vi "12kW_SubVI.vi"() -> ()   [LabVIEW 2020]
panel:
  out "Step 7\nIndicator":bool
  out "Step 4\nIndicator":bool
  out "Step 10\nIndicator":bool
  out "Step 9\nIndicator":bool
  out "Step 8\nIndicator":bool
  out "Step 6\nIndicator":bool
  out "Step 5\nIndicator":bool
  out "Step 3\nIndicator":bool
  out "Step 2\nIndicator":bool
  out "Step 1\nIndicator":bool
  in  "Stop":bool
  out "Voltage (V)":dbl
  in  "Power Supply":bool
  out "B":bool
  out "Y":bool
  out "R":bool
  out "No. of Resistors Used":i32
  in  "Step Type":enum32{"Variable Steps", "Equal Steps"}(tab)
  in  "Step 1\n250W":bool
  in  "Step 2\n250W":bool
  in  "Step 3\n500W":bool
  in  "Step 4\n1000W":bool
  in  "Step 5\n1000W":bool
  in  "Step 6\n1000W":bool
  in  "Step 7\n2000W":bool
  in  "Step 8\n2000W":bool
  in  "Step 9\n2000W":bool
  in  "Step 10\n2000W":bool
  in  "No. of Equal Steps":T1(tab)
  in  "Step 2\n6000W":bool
  in  "Step 1\n6000W":bool
  in  "Step 3\n4000W":bool
  in  "Step 2\n4000W":bool
  in  "Step 1\n4000W":bool
  in  "Step 4\n3000W":bool
  in  "Step 3\n3000W":bool
  in  "Step 2\n3000W":bool
  in  "Step 1\n3000W":bool
  in  "Step 6\n2000W":bool
  in  "Step 5\n2000W":bool
  in  "Step 4\n2000W":bool
  in  "Step 3\n2000W":bool
  in  "Step 2\n2000W":bool
  in  "Step 1\n2000W":bool
  in  "Master Switch":bool
  out "Load (kW)":dbl
  out "Current (A)":dbl format="%.4f"
  # "Three Phase Variable Resistive Load Bank with 12kW Maximum Capacity and 10 Step Control"
  # "690 ohm\n0.35 A"
  # "All resistors are connected in 3 phase star formation"
  # "690 ohm\n0.35 A"
  # "344 ohm\n0.70 A"
  # "3 Phase Voltage Indicator"
  # "172 ohm\n1.39 A"
  # "172 ohm\n1.39 A"
  # "172 ohm\n1.39 A"
  # "86 ohm\n2.78 A"
  # "86 ohm\n2.78 A"
  # "86 ohm\n2.78 A"
  # "Each Resistor Looks Like This"
  # "86 ohm\n2.78 A"
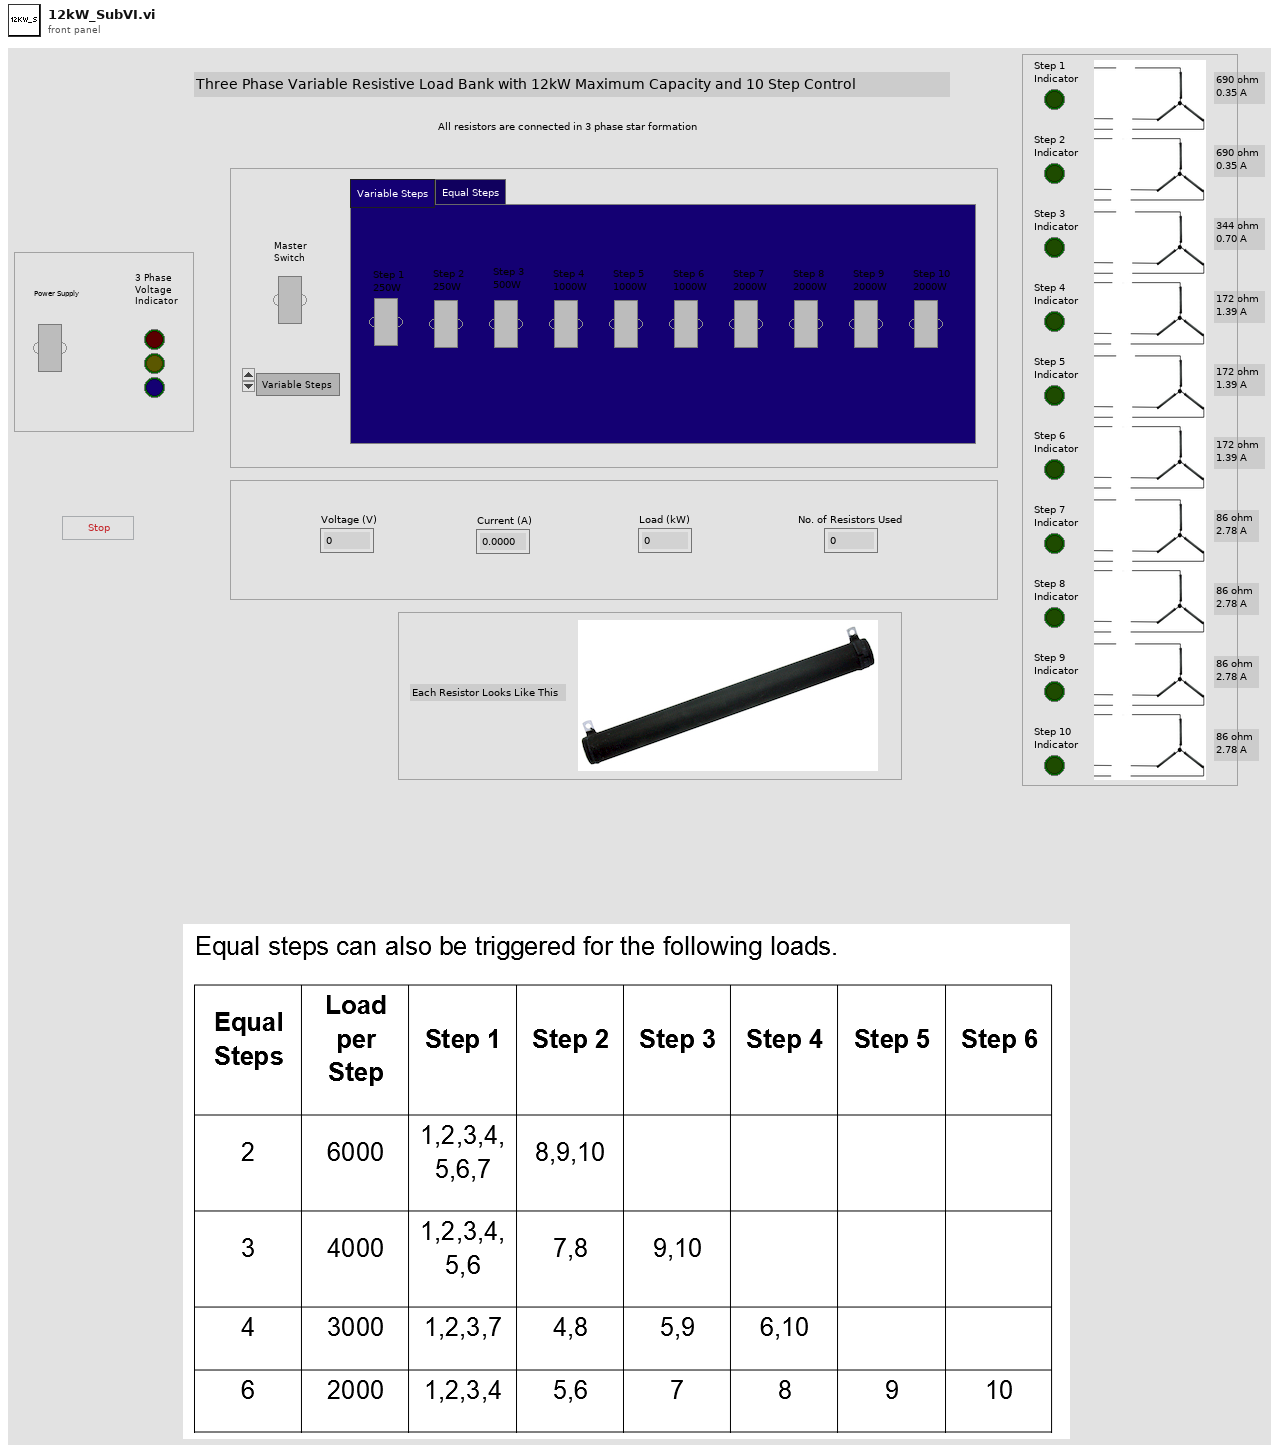
[diagram p1: front panel]
types:
  T1 = enum32{"2 Steps", "3 Steps", "4 Steps", "6 Steps"}
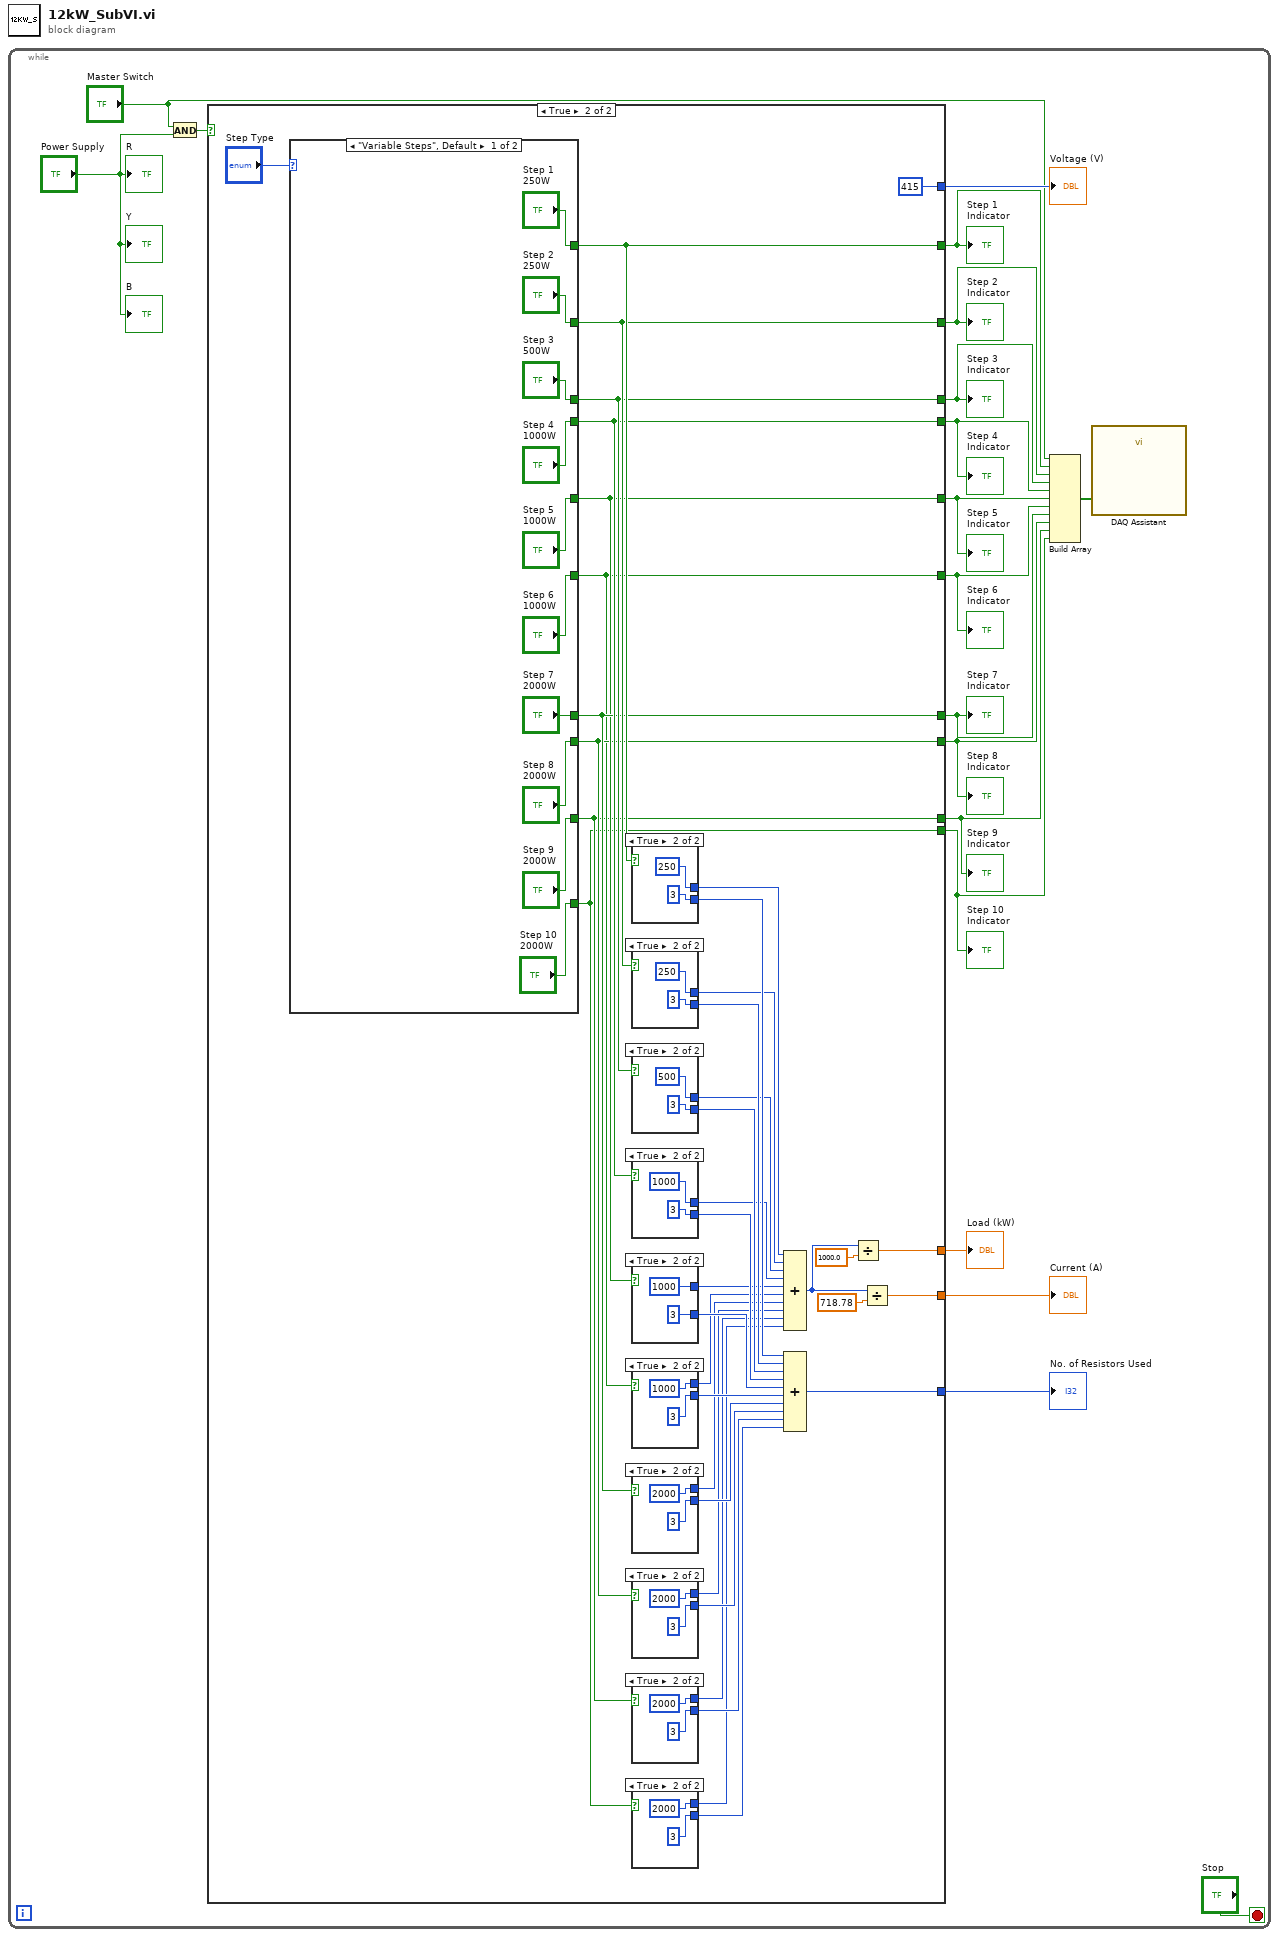
[diagram p0: block diagram]
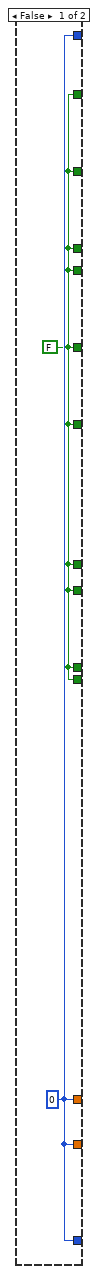
[diagram p2: hidden frame]
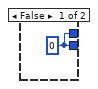
[diagram p3: hidden frame]
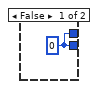
[diagram p4: hidden frame]
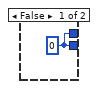
[diagram p5: hidden frame]
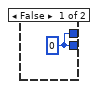
[diagram p6: hidden frame]
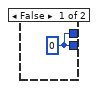
[diagram p7: hidden frame]
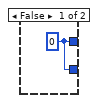
[diagram p8: hidden frame]
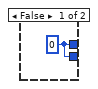
[diagram p9: hidden frame]
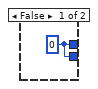
[diagram p10: hidden frame]
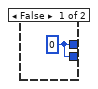
[diagram p11: hidden frame]
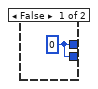
[diagram p12: hidden frame]
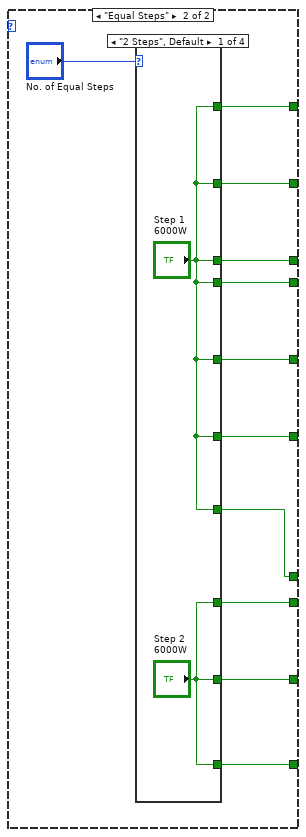
[diagram p13: hidden frame]
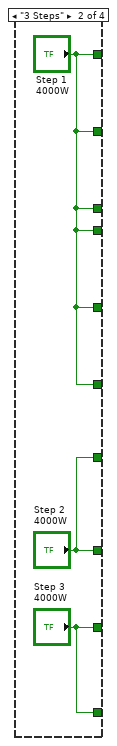
[diagram p14: hidden frame]
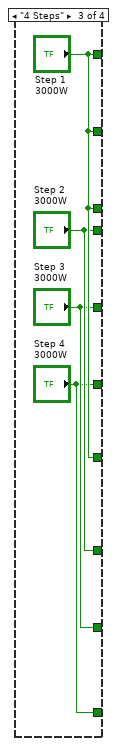
[diagram p15: hidden frame]
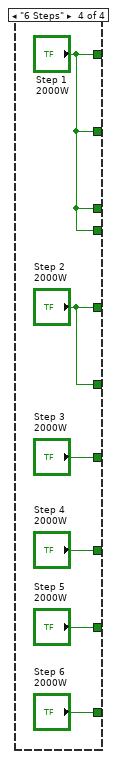
[diagram p16: hidden frame]
diagram:
  n1 = while {
    stop <- "Stop" stop-if-true
    n2 = And(x="Master Switch", y="Power Supply") -> (x .and. y?=w15:bool)
    n3 = case shown="True" w15 {
      tunnel: [w21 w36] -> w18
      tunnel: [w21 w32] -> w17
      tunnel: [w21 w33] -> w19
      tunnel: [w21 415] -> w16
      tunnel: [w20 w31] -> w3
      tunnel: [w20 w30] -> w4
      tunnel: [w20 w29] -> w5
      tunnel: [w20 w28] -> w6
      tunnel: [w20 w27] -> w7
      tunnel: [w20 w26] -> w1
      tunnel: [w20 w25] -> w8
      tunnel: [w20 w24] -> w2
      tunnel: [w20 w23] -> w9
      tunnel: [w20 w22] -> w10
      frame False {
        w20 = FALSE
        w21 = 0
      }
      frame True {
        n4 = case shown="\"Variable Steps\", Default" "Step Type" {
          tunnel: ["Step 10\n2000W" w100] -> w22
          tunnel: ["Step 9\n2000W" w101] -> w23
          tunnel: ["Step 8\n2000W" w102] -> w25
          tunnel: ["Step 7\n2000W" w103] -> w27
          tunnel: ["Step 6\n1000W" w104] -> w24
          tunnel: ["Step 5\n1000W" w105] -> w26
          tunnel: ["Step 4\n1000W" w106] -> w28
          tunnel: ["Step 3\n500W" w107] -> w29
          tunnel: ["Step 2\n250W" w108] -> w30
          tunnel: ["Step 1\n250W" w109] -> w31
          frame "Variable Steps", Default {
          }
          frame "Equal Steps" {
            n5 = case shown="\"2 Steps\", Default" "No. of Equal Steps" {
              tunnel: ["Step 1\n6000W" "Step 1\n4000W" "Step 1\n3000W" "Step 1\n2000W"] -> w109
              tunnel: ["Step 1\n6000W" "Step 1\n4000W" "Step 1\n3000W" "Step 1\n2000W"] -> w108
              tunnel: ["Step 1\n6000W" "Step 1\n4000W" "Step 1\n3000W" "Step 1\n2000W"] -> w107
              tunnel: ["Step 1\n6000W" "Step 1\n4000W" "Step 2\n3000W" "Step 1\n2000W"] -> w106
              tunnel: ["Step 1\n6000W" "Step 1\n4000W" "Step 3\n3000W" "Step 2\n2000W"] -> w105
              tunnel: ["Step 1\n6000W" "Step 1\n4000W" "Step 4\n3000W" "Step 2\n2000W"] -> w104
              tunnel: ["Step 1\n6000W" "Step 2\n4000W" "Step 1\n3000W" "Step 3\n2000W"] -> w103
              tunnel: ["Step 2\n6000W" "Step 2\n4000W" "Step 2\n3000W" "Step 4\n2000W"] -> w102
              tunnel: ["Step 2\n6000W" "Step 3\n4000W" "Step 3\n3000W" "Step 5\n2000W"] -> w101
              tunnel: ["Step 2\n6000W" "Step 3\n4000W" "Step 4\n3000W" "Step 6\n2000W"] -> w100
              frame "2 Steps", Default {
              }
              frame "3 Steps" {
              }
              frame "4 Steps" {
              }
              frame "6 Steps" {
              }
            }
          }
        }
        n6 = case shown="True" w31 {
          tunnel: [w87 250] -> w37
          tunnel: [w87 3] -> w47
          frame False {
            w87 = 0
          }
          frame True {
          }
        }
        n7 = case shown="True" w30 {
          tunnel: [w84 250] -> w38
          tunnel: [w84 3] -> w48
          frame False {
            w84 = 0
          }
          frame True {
          }
        }
        n8 = case shown="True" w29 {
          tunnel: [w81 500] -> w39
          tunnel: [w81 3] -> w49
          frame False {
            w81 = 0
          }
          frame True {
          }
        }
        n9 = case shown="True" w28 {
          tunnel: [w78 1000] -> w40
          tunnel: [w78 3] -> w50
          frame False {
            w78 = 0
          }
          frame True {
          }
        }
        n10 = case shown="True" w26 {
          tunnel: [w75 1000] -> w41
          tunnel: [w75 3] -> w51
          frame False {
            w75 = 0
          }
          frame True {
          }
        }
        n11 = case shown="True" w24 {
          tunnel: [w72 1000] -> w42
          tunnel: [w72 3] -> w52
          frame False {
            w72 = 0
          }
          frame True {
          }
        }
        n12 = case shown="True" w27 {
          tunnel: [w69 2000] -> w43
          tunnel: [w69 3] -> w53
          frame False {
            w69 = 0
          }
          frame True {
          }
        }
        n13 = case shown="True" w25 {
          tunnel: [w66 2000] -> w44
          tunnel: [w66 3] -> w54
          frame False {
            w66 = 0
          }
          frame True {
          }
        }
        n14 = case shown="True" w23 {
          tunnel: [w63 2000] -> w45
          tunnel: [w63 3] -> w55
          frame False {
            w63 = 0
          }
          frame True {
          }
        }
        n15 = case shown="True" w22 {
          tunnel: [w60 2000] -> w46
          tunnel: [w60 3] -> w56
          frame False {
            w60 = 0
          }
          frame True {
          }
        }
        n16 = Compound Arithmetic op=ADD(w37, w38, w39, w40, w41, w42, w43, w44, w45, w46) -> (w35:i32)
        n17 = Compound Arithmetic op=ADD(w47, w48, w49, w50, w51, w52, w53, w54, w55, w56) -> (w36:i32)
        n18 = Divide(x=w35, y=1000.0) -> (x/y=w33:dbl)
        n19 = Divide(x=w35, y=718.78) -> (x/y=w32:dbl)
      }
    }
    "Load (kW)" <- w19
    "Current (A)" <- w17
    "No. of Resistors Used" <- w18
    "Voltage (V)" <- w16
    "Step 1\nIndicator" <- w3
    "Step 2\nIndicator" <- w4
    "Step 3\nIndicator" <- w5
    "Step 4\nIndicator" <- w6
    "Step 7\nIndicator" <- w7
    "Step 5\nIndicator" <- w1
    "Step 8\nIndicator" <- w8
    "Step 6\nIndicator" <- w2
    "Step 9\nIndicator" <- w9
    "Step 10\nIndicator" <- w10
    n20 = Build Array("Master Switch", w3, w4, w5, w6, w1, w2, w7, w8, w9, w10) -> (w13:bool[])
    n21 = call "DAQ Assistant"("data"=w13) -> ()  [unwired: 17 in, 2 out]
    "B" <- "Power Supply"
    "Y" <- "Power Supply"
    "R" <- "Power Supply"
  }
